vi "Write Test Context.vi"(8 "error in (no error)":errorcluster, 10 "Test Context":T1, 11 "Sequence Engine in":refnum<class "Sequence Engine.lvclass">) -> (0 "error out":errorcluster, 3 "Sequence Engine out":refnum<class "Sequence Engine.lvclass">)   [LabVIEW 2021, in "Sequence Engine.lvlib" / "Sequence Engine.lvclass"]
uses:
  Sequence Engine.lvclass
  Sequence Context.ctl
  Sequence Engine.lvclass/Sequence Engine.ctl
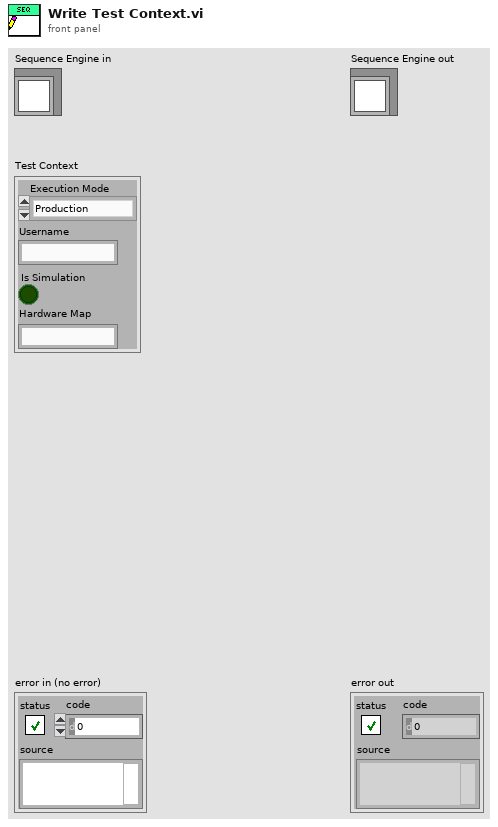
[diagram p1: front panel]
types:
  T1 = typedef "Sequence Engine.lvlib/Sequence Engine.lvclass/Sequence Context.ctl" = cluster{"Execution Mode":enum16{"Production", "MSA1", "Trial"}, "Username":string, "Is Simulation":bool, "Hardware Map":string}
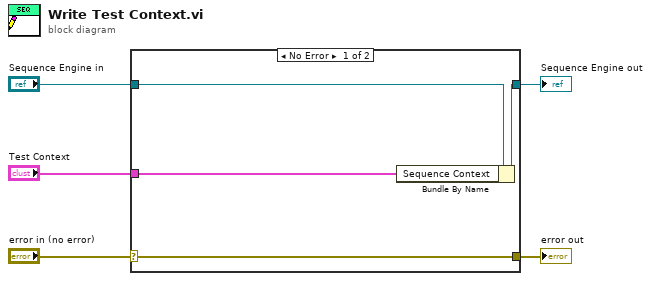
[diagram p0: block diagram]
diagram:
  n1 = case shown="No Error" "error in (no error)" {
    selector: "error in (no error)" -> [w9 w10]
    tunnel: [w9 w10] -> w4
    tunnel: [w7 w11] -> w2
    tunnel: "Sequence Engine in" -> [w8 w11]
    tunnel: "Test Context" -> [w6 _]
    frame No Error {
      n2 = Bundle By Name(cluster=w8, "Sequence Context"=w6) -> (w7:refnum<class "Sequence Engine.lvclass">)
    }
    frame Error {
    }
  }
  "error out" <- w4
  "Sequence Engine out" <- w2
